vi "SmoothVelocity.vi"(8 "polynomial order":i32=1, 9 "side points":i32=15, 10 "Velocity field":csg[][][](array[numeric])) -> (2 "Out":csg[][][](array[numeric]))   [LabVIEW 2022 SP3]
uses:
  <vilib>/Analysis/3filter.llb/Savitzky-Golay Filter (DBL).vi
  <vilib>/Analysis/NI_AALBase.lvlib
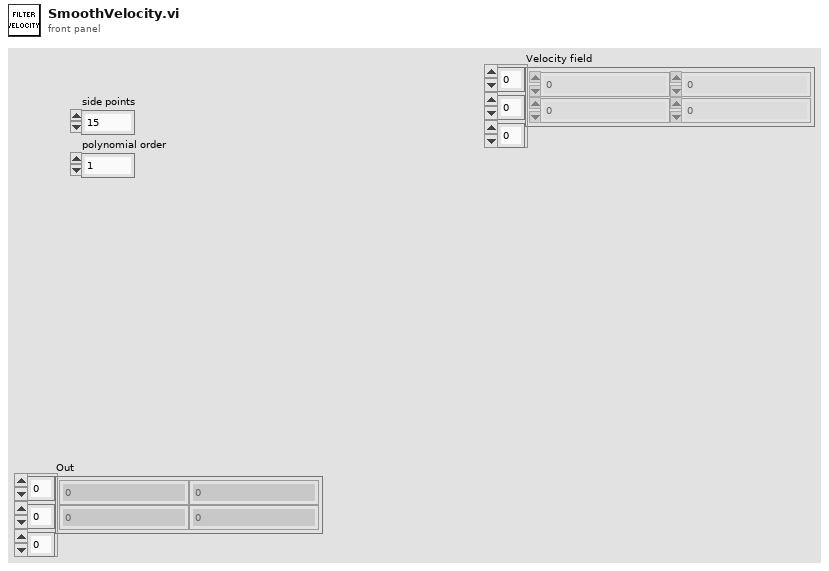
[diagram p1: front panel]
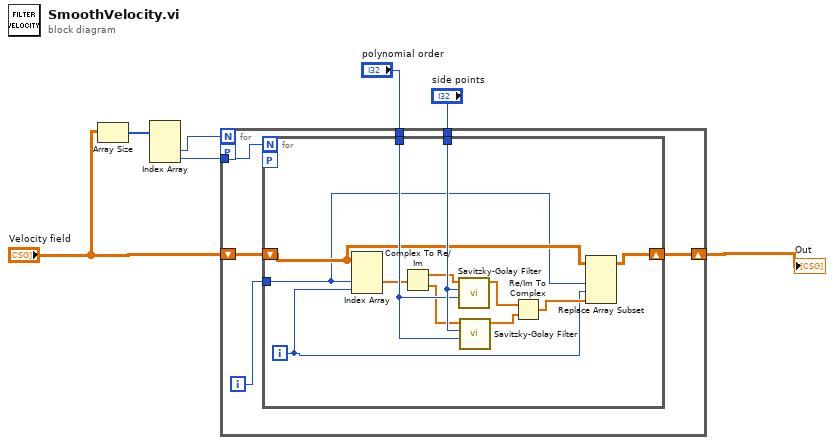
[diagram p0: block diagram]
diagram:
  n1 = Array Size(array="Velocity field") -> (size(s)=w3:i32[])
  n2 = Index Array(array=w3) -> (element #2=w1:i32, element #3=w2:i32)  [unwired: 3 in, 1 out]
  n3 = for {
    N: w1 -> [_]
    tunnel: "side points" -> [w11]
    tunnel: "polynomial order" -> [w10]
    shift-right: [w9] -> w5
    shift-left: "Velocity field" -> [w13]
    tunnel: w2 -> [w8]
    workers-P: _ -> [_]
    i -> [w12]
    n4 = for {
      N: w8 -> [_]
      tunnel: w12 -> [w14]
      tunnel: w11 -> [w25]
      tunnel: w10 -> [w24]
      shift-right: [w18] -> w9
      shift-left: w13 -> [w17]
      workers-P: _ -> [_]
      i -> [w15]
      n5 = Index Array(array=w17, index (dim 1)=w14, index (dim 2)=w15) -> (element=w23:csg[])  [unwired: 1 in]
      n6 = Complex To Re/Im(x + iy=w23) -> (x=w21:sgl[], y=w22:sgl[])
      n7 = call-poly <vilib>:"Savitzky-Golay Filter.vi"("polynomial order"=w24, "side points"=w25, "X"=w21) -> ("Filtered X"=w20:dbl[])  [unwired: 7 in, 1 out]
      n8 = call-poly <vilib>:"Savitzky-Golay Filter.vi"("polynomial order"=w24, "side points"=w25, "X"=w22) -> ("Filtered X"=w19:dbl[])  [unwired: 7 in, 1 out]
      n9 = Re/Im To Complex(1:w19, 2:w20) -> (0:w16:cdb[])
      n10 = Replace Array Subset(array=w17, new element=w16, index (dim 1)=w14, index (dim 2)=w15) -> (w18:csg[][][])  [unwired: 1 in]
    }
  }
  "Out" <- w5
